vi "Simple TCP - Client.vi"() -> ()   [LabVIEW 2019]
doc: "Demonstrates how to open a connection to an TCP server, read the data being sent, and display the data on a chart. This VI is designed to stop if the TCP connection is terminated."
panel:
  out "Current Alt":dbl
  in  "Server Closed":string="The server VI closed the connection."
  out "Waveform Graph":dbl[](graph)
  in  "Stop":bool
  # "Overview: Demonstrates the use of the TCP functions to connect to a TCP server VI and receive data.\nInstructions:\n1. Ensure Simple TCP - Server.vi is already running.\n2. Run the VI.\n3. Click Stop to stop the VI. Note that if you stop the server VI, this VI will stop automatically."
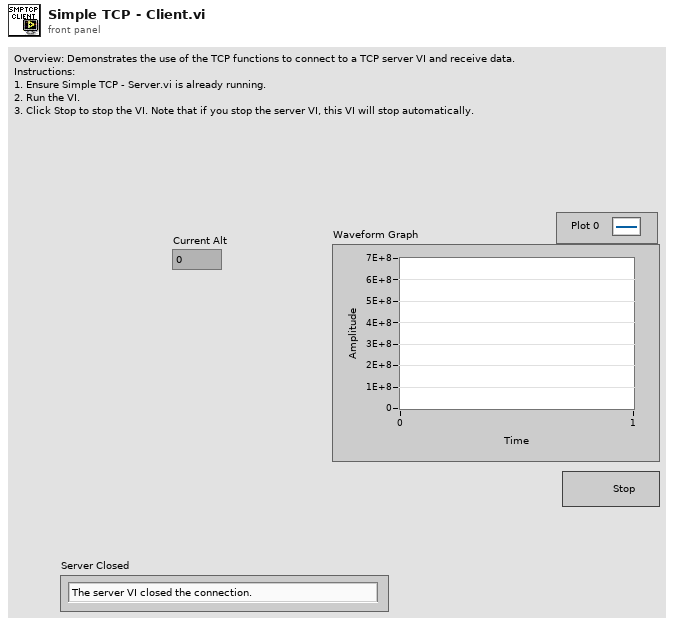
[diagram p1: front panel]
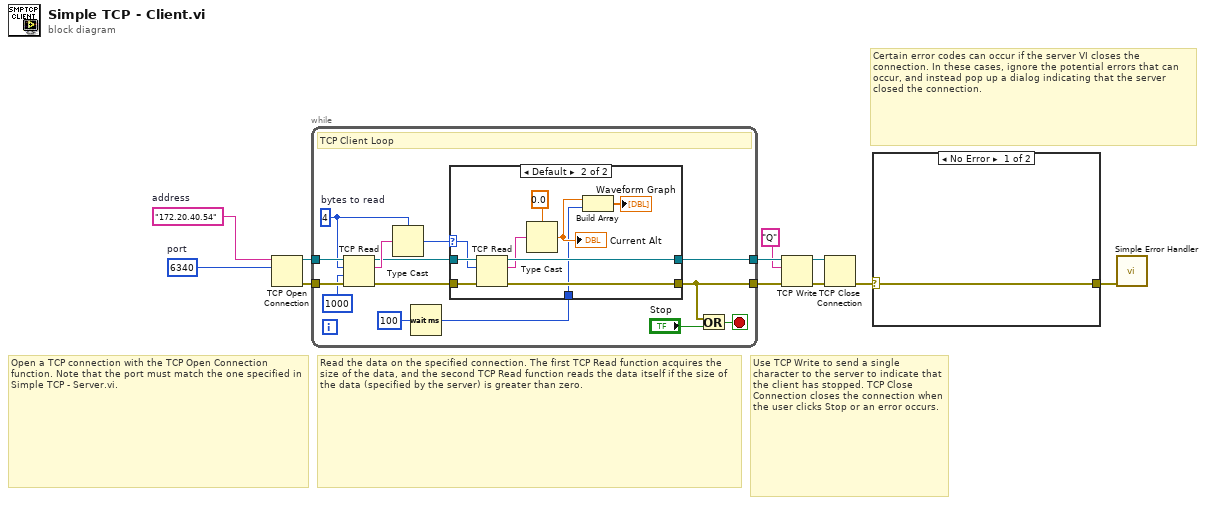
[diagram p0: block diagram]
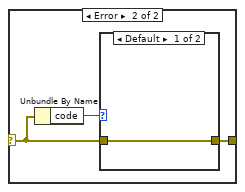
[diagram p2: hidden frame]
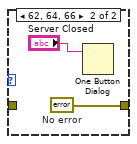
[diagram p3: hidden frame]
diagram:
  w1 = u16 6340  # port
  w2 = "172.20.40.54"  # address
  # "Certain error codes can occur if the server VI closes the connection. In these cases, ignore the potential errors that can occur, and instead pop up a dialog indicating that the server closed the connection."
  # "Use TCP Write to send a single character to the server to indicate that the client has stopped. TCP Close Connection closes the connection when the user clicks Stop or an error occurs."
  # "Read the data on the specified connection. The first TCP Read function acquires the size of the data, and the second TCP Read function reads the data itself if the size of the data (specified by the server) is greater than zero."
  # "Open a TCP connection with the TCP Open Connection function. Note that the port must match the one specified in Simple TCP - Server.vi."
  n1 = TCP Open Connection(address=w2, remote port or service name=w1) -> (connection ID=w11:refnum<k5>, error out=w10:errorcluster)  [unwired: 3 in]
  n2 = while {
    tunnel: w10 -> [w21]
    tunnel: w11 -> [w22]
    tunnel: [w16] -> w8
    tunnel: [w15] -> w6
    stop <- w18 stop-if-true
    w20 = 4  # bytes to read
    # "TCP Client Loop"
    n3 = TCP Read(connection ID=w22, bytes to read=w20, error in (no error)=w21, 9:1000 ("timeout ms (25000)")) -> (connection ID out=w24:refnum<k5>, data out=w25:string, error out=w23:errorcluster)  [unwired: 1 in]
    n4 = Type Cast(type=w20, x=w25) -> (*(type *) &x=w14:i32)
    n5 = Wait (ms)(milliseconds to wait=u32 100) -> (millisecond timer value=w12:u32)
    n6 = case shown="Default" w14 {
      selector: w14 -> [_ w31]
      tunnel: w24 -> [w27 w37]
      tunnel: w23 -> [w26 w36]
      tunnel: [w27 w34] -> w16
      tunnel: [w26 w33] -> w15
      tunnel: w12 -> [_ w29]
      frame ..0 {
        # "The server has not written any data"
      }
      frame Default {
        n7 = TCP Read(connection ID=w37, bytes to read=w31, error in (no error)=w36) -> (connection ID out=w34:refnum<k5>, data out=w32:string, error out=w33:errorcluster)  [unwired: 2 in]
        n8 = Type Cast(type=0.0 ("chart"), x=w32) -> (*(type *) &x=w30:dbl)
        "Current Alt" <- w30
        n9 = Build Array(w30, w29) -> (→"Waveform Graph":dbl[])
      }
    }
    n10 = Or(x=w15, y="Stop") -> (x .or. y?=w18:bool)
  }
  n11 = TCP Write(connection ID=w8, data in="Q", error in (no error)=w6) -> (connection ID out=w9:refnum<k5>, error out=w7:errorcluster)  [unwired: 2 out]
  n12 = TCP Close Connection(connection ID=w9, error in (no error)=w7) -> (error out=w4:errorcluster)  [unwired: 1 in, 1 out]
  n13 = case shown="No Error" w4 {
    selector: w4 -> [w38 w40]
    tunnel: [w38 w39] -> w3
    frame No Error {
    }
    frame Error {
      n14 = Unbundle By Name(w40) -> ("code"=w41:i32)
      n15 = case shown="Default" w41 {
        tunnel: w40 -> [w42 _]
        tunnel: [w42 w44] -> w39
        frame Default {
        }
        frame 62, 64, 66 {
          w44 = errorcluster {"status"=FALSE, "code"=0, "source"=""}  # No error
          n16 = One Button Dialog(message="Server Closed") -> ()  [unwired: 1 in, 1 out]
        }
      }
    }
  }
  n17 = call <vilib>:"Simple Error Handler.vi"("error in (no error)"=w3) -> ()  [unwired: 4 in, 5 out]
